vi "PXI-Channel Index to Physical Channel-1056.vi"(10 "index":i32) -> (2 "element":tag)   [LabVIEW 2020]
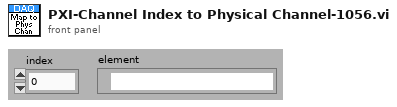
[diagram p1: front panel]
types:
  T1 = cluster{"DAQChan to PhysDev":i32[][], "PhysDev to DAQChan":i32[][]}
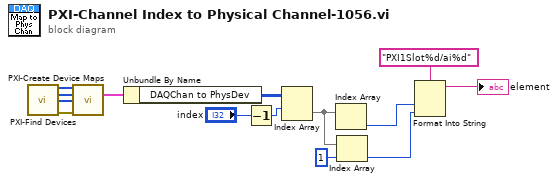
[diagram p0: block diagram]
diagram:
  n1 = call "PXI-Find Devices.vi"() -> ("Num AO"=w12:i32[], "Num AI"=w11:i32[], "Slot Num"=w14:u32[], "error out"=w13:errorcluster)  [unwired: 12 in]
  n2 = call "PXI-Create Device Maps.vi"("Num AO"=w12, "Num AI"=w11, "Slot Num"=w14, "error in (no error)"=w13) -> ("AI Map"=w10:T1)  [unwired: 9 in, 2 out]
  n3 = Unbundle By Name(w10) -> ("DAQChan to PhysDev"=w9:i32[][])
  n4 = Decrement(x="index") -> (x-1=w1:i32)
  n5 = Index Array(array=w9, index (row)=w1) -> (element=w7:i32[])  [unwired: 1 in]
  n6 = Index Array(array=w7) -> (element=w4:i32)  [unwired: 1 in]
  n7 = Index Array(array=w7, index=1) -> (element=w3:i32)
  n8 = Format Into String(format string="PXI1Slot%d/ai%d", w4, w3) -> (resulting string=→"element":string)  [unwired: 2 in, 1 out]
